vi "Parser_0x55_(SubVI).vi"(11 "String in":string) -> (2 "CheckSumGood":bool, 3 "Cluster":T1)   [LabVIEW 2017, in "LV_Unicorn.lvlib"]
uses:
  LV_Unicorn.lvlib
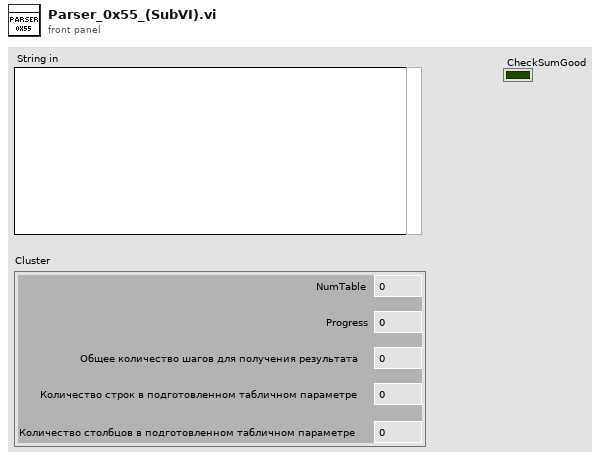
[diagram p1: front panel]
types:
  T1 = cluster{"NumTable":i32, "Progress":i32, "Общее количество шагов для получения результата":i32, "Количество строк в подготовленном табличном параметре":i32, "Количество столбцов в подготовленном табличном параметре":i32}
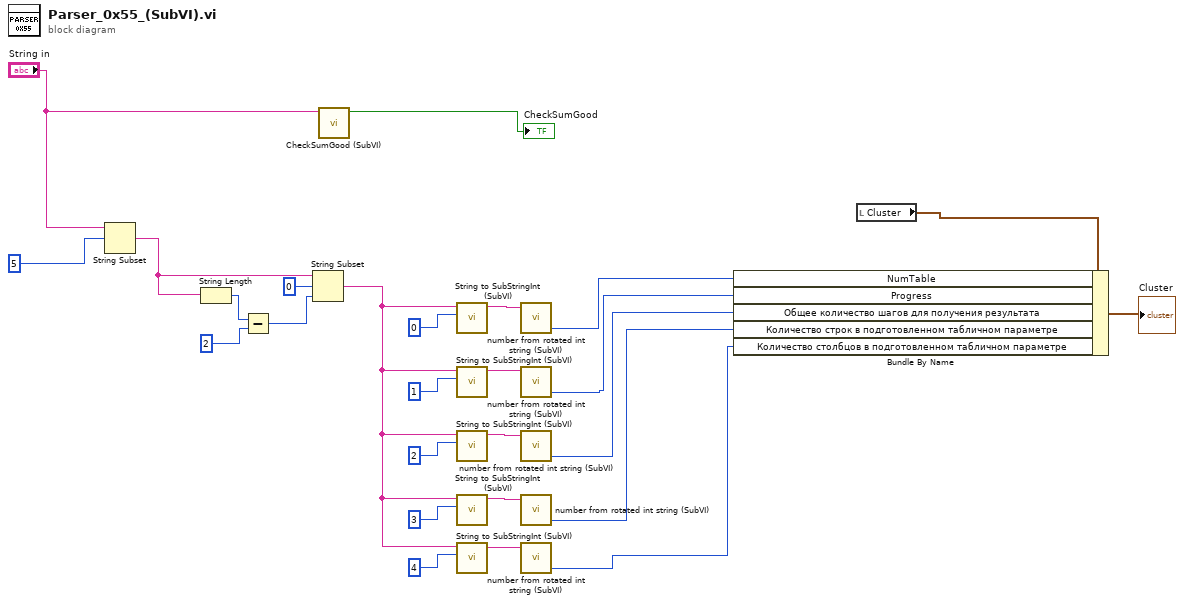
[diagram p0: block diagram]
diagram:
  n1 = String Subset(string="String in", offset (0)=5) -> (substring=w15:string)  [unwired: 1 in]
  n2 = String Length(string=w15) -> (length=w19:i32)
  n3 = Subtract(x=w19, y=2) -> (x-y=w16:i32)
  n4 = String Subset(string=w15, offset (0)=0, length (rest)=w16) -> (substring=w10:string)
  n5 = call "CheckSumGood (SubVI).vi"("String in"="String in") -> ("CheckSumGood"=→"CheckSumGood":bool)  [unwired: 10 in]
  n6 = call "String to SubStringInt (SubVI).vi"("Nx4byte"=u32 0, "String in in"=w10) -> ("String out"=w21:string)  [unwired: 9 in]
  n7 = call "String to SubStringInt (SubVI).vi"("Nx4byte"=u32 1, "String in in"=w10) -> ("String out"=w22:string)  [unwired: 9 in]
  n8 = call "String to SubStringInt (SubVI).vi"("Nx4byte"=u32 2, "String in in"=w10) -> ("String out"=w26:string)  [unwired: 9 in]
  n9 = call "String to SubStringInt (SubVI).vi"("Nx4byte"=u32 3, "String in in"=w10) -> ("String out"=w13:string)  [unwired: 9 in]
  n10 = call "String to SubStringInt (SubVI).vi"("Nx4byte"=u32 4, "String in in"=w10) -> ("String out"=w11:string)  [unwired: 9 in]
  n11 = call "number from rotated int string (SubVI).vi"("String"=w21) -> ("int number"=w5:i32)  [unwired: 2 in, 2 out]
  n12 = call "number from rotated int string (SubVI).vi"("String"=w22) -> ("int number"=w4:i32)  [unwired: 2 in, 2 out]
  n13 = call "number from rotated int string (SubVI).vi"("String"=w26) -> ("int number"=w3:i32)  [unwired: 2 in, 2 out]
  n14 = call "number from rotated int string (SubVI).vi"("String"=w13) -> ("int number"=w2:i32)  [unwired: 2 in, 2 out]
  n15 = call "number from rotated int string (SubVI).vi"("String"=w11) -> ("int number"=w1:i32)  [unwired: 2 in, 2 out]
  n16 = local read "Cluster"() -> (w7:T1)
  n17 = Bundle By Name(cluster=w7, "NumTable"=w5, "Progress"=w4, "Общее количество шагов для получения результата"=w3, "Количество строк в подготовленном табличном параметре"=w2, "Количество столбцов в подготовленном табличном параметре"=w1) -> (→"Cluster":T1)
